vi "Filtered Noise.vi"(1 "amplitude: A":dbl=1.0 format="%.2f") -> (0 "filtered noise":dbl format="%.2f")   [LabVIEW 2023]
doc: "Generates random numbers with a little bit of smoothing and selectable amplitude."
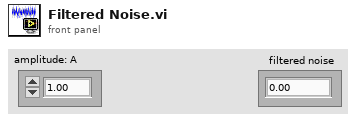
[diagram p1: front panel]
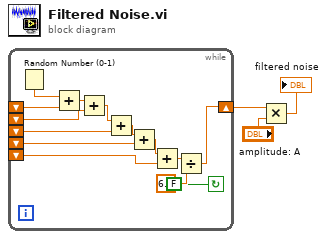
[diagram p0: block diagram]
diagram:
  n1 = while {
    shift-left: _ -> [w14]
    shift-left: _ -> [w13]
    shift-left: _ -> [w12]
    shift-left: _ -> [w11]
    shift-left: _ -> [w17]
    shift-right: [w5] -> w3
    stop <- FALSE continue-if-true
    n2 = Random Number (0-1)() -> (number: 0 to 1=w16:dbl)
    n3 = Add(x=w16, y=w17) -> (x+y=w15:dbl)
    n4 = Add(x=w15, y=w14) -> (x+y=w10:dbl)
    n5 = Add(x=w10, y=w13) -> (x+y=w9:dbl)
    n6 = Add(x=w9, y=w12) -> (x+y=w8:dbl)
    n7 = Add(x=w8, y=w11) -> (x+y=w7:dbl)
    n8 = Divide(x=w7, y=6.0) -> (x/y=w5:dbl)
  }
  n9 = Multiply(x=w3, y="amplitude: A") -> (x*y=→"filtered noise":dbl)
